vi "encodeStream.vi"(8 "error in (no error)":errorcluster, 11 "tBSONBoolean in":refnum<class "tBSONBoolean.lvclass">) -> (0 "error out":errorcluster, 2 "Byte Array":u8[](array[numeric]), 3 "tBSONBoolean out":refnum<class "tBSONBoolean.lvclass">)   [LabVIEW 2013, in "BSON.lvlib" / "tBSONBoolean.lvclass"]
uses:
  tBSONBoolean.lvclass
  tBSONElement/tBSONElement.lvclass
  getValue.vi
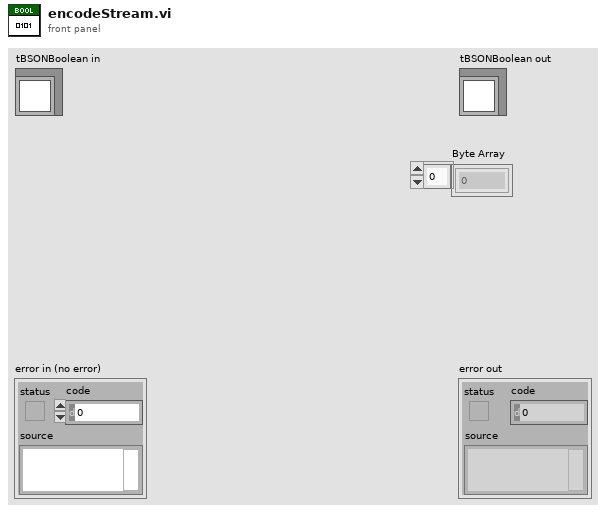
[diagram p1: front panel]
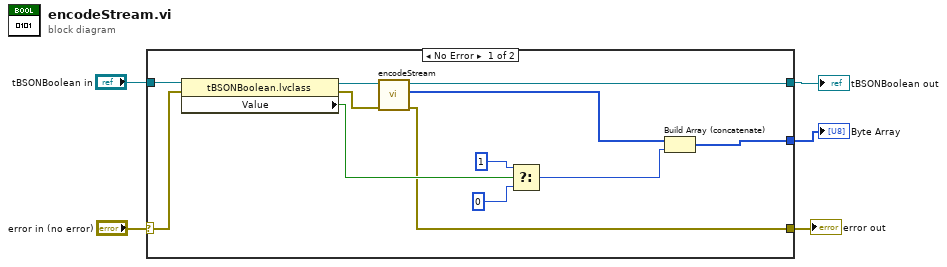
[diagram p0: block diagram]
diagram:
  n1 = case shown="No Error" "error in (no error)" {
    selector: "error in (no error)" -> [w16 w18]
    tunnel: "tBSONBoolean in" -> [w17 w19]
    tunnel: [w7 w19] -> w5
    tunnel: [w8 w18] -> w3
    tunnel: [w15 _] -> w1
    frame No Error {
      n2 = property class="tBSONBoolean.lvclass"(reference=w17, error in=w16) -> (reference out=w10:refnum<class "tBSONBoolean.lvclass">, error out=w9:errorcluster, "Value"=w12:bool)
      n3 = call-parent "encodeStream.vi"("error in (no error)"=w9, "tBSONElement in"=w10) -> ("error out"=w8:errorcluster, "Byte Array"=w6:u8[], "tBSONElement out"=w7:refnum<class "tBSONBoolean.lvclass">)  [unwired: 7 in]
      n4 = Select(t=u8 1, s=w12, f=u8 0) -> (s? t:f=w11:u8)
      n5 = Build Array (concatenate)(w6, w11) -> (w15:u8[])
    }
    frame Error {
    }
  }
  "error out" <- w3
  "tBSONBoolean out" <- w5
  "Byte Array" <- w1
